vi "ReadChannelStatusFPGA.vi"(7 "IEPE settling blocks":i32=20, 8 "error in":errorcluster, 10 "Wfm Data":waveform(sgl)[](array[waveform]), 11 "Dynamic FPGA VI Reference":T1) -> (0 "error out":errorcluster, 2 "Wfm Data":waveform(sgl)[](array[waveform]), 3 "Dynamic FPGA VI Reference":T1)   [LabVIEW 2015]
doc: "This VI sets the host application's data buffer size, which is critical for maximum data throughput. This buffer is responsible for receiving data coming from the FPGA DMA FIFO. For the continuous case the buffer size should be many times larger than your read size. In the finite case, the timing VIs automatically call this VI and set the buffer size equal to the number of samples in the acquisition."
uses:
  <vilib>/addons/InsightCM/Devices/Shared/cRIOWfmAcq/subVIs/RIO Wfm Cust Ctrls/rwfm_DynamicFPGAref2.ctl
  <vilib>/addons/InsightCM/Devices/Shared/cRIOWfmAcq/subVIs/stretchState.ctl
  <vilib>/rvi/interface/nirviReadWriteControl/nirviReadWriteControl.xnode
  <vilib>/addons/InsightCM/Devices/Shared/cRIOWfmAcq/cRIOWfmLib.lvlib
  NiFpgaLv.dll
  <vilib>/Utility/error.llb/Error Cluster From Error Code.vi
  <vilib>/rvi/interface/Simulation/niFpgaSimulationCallBeginRW.vi
  <vilib>/rvi/errors/niLvFpgaAdjustHostInterfaceError.vi
  <vilib>/addons/InsightCM/Utilities/ChannelStatus/ChannelStatus.lvlib
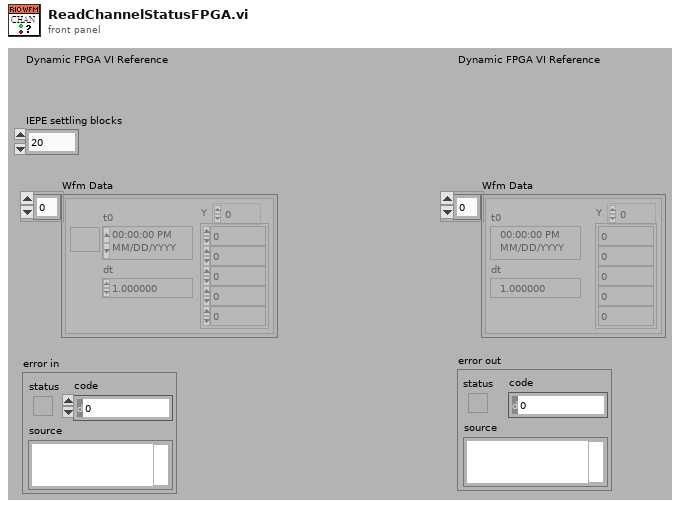
[diagram p1: front panel]
types:
  T1 = typedef "cRIOWfmLib.lvlib/rwfm_DynamicFPGAref2.ctl" = refnum<k20>
  T2 = typedef "cRIOWfmLib.lvlib/stretchState.ctl" = cluster{"input":bool, "output":bool, "pulse count":i32}
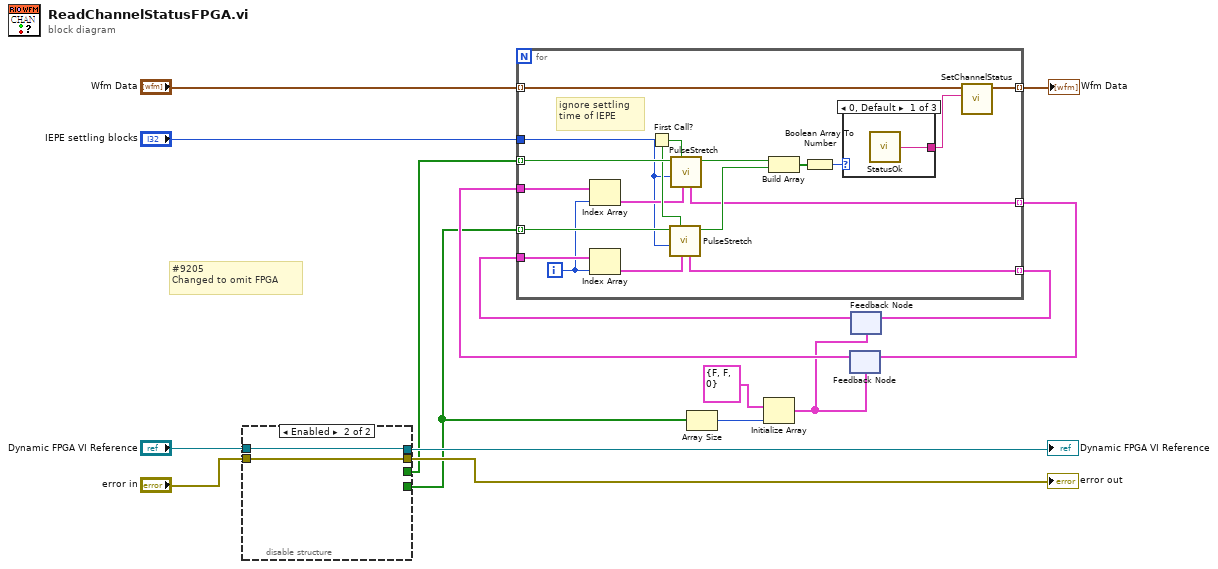
[diagram p0: block diagram]
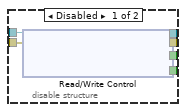
[diagram p2: hidden frame]
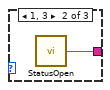
[diagram p3: hidden frame]
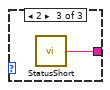
[diagram p4: hidden frame]
diagram:
  # "#9205\nChanged to omit FPGA"
  n1 = disable-structure shown="Enabled" {
    disable-tunnel: "Dynamic FPGA VI Reference" -> [w22 w24]
    disable-tunnel: "error in" -> [w21 w23]
    disable-tunnel: [w20 w24] -> w14
    disable-tunnel: [w19 w23] -> w13
    disable-tunnel: [w18 _] -> w11
    disable-tunnel: [w17 _] -> w5
    frame Disabled {
      n2 = xnode "Read/Write Control"("FPGA VI Reference In"=w22, "error in"=w21) -> ("FPGA VI Reference Out"=w20:T1, "error out"=w19:errorcluster, "Open Loop Chan Array"=w18:bool[], "Short Circuit Chan Array"=w17:bool[])
    }
    frame Enabled {
    }
  }
  "error out" <- w13
  "Dynamic FPGA VI Reference" <- w14
  n3 = Array Size(array=w5) -> (size(s)=w4:i32)
  n4 = Initialize Array(T2 {"input"=FALSE, "output"=FALSE, "pulse count"=0} ("element"), w4) -> (w2:T2[])
  n5 = feedback #1(w2) -> (w6:T2[])
  n6 = feedback #2(w2) -> (w8:T2[])
  n7 = for {
    tunnel: "Wfm Data" -> [w26] mode=indexing
    tunnel: w11 -> [w42] mode=indexing
    tunnel: w5 -> [w40] mode=indexing
    tunnel: [w25] -> w10 mode=indexing
    tunnel: [w37] -> w9 mode=indexing
    tunnel: [w36] -> w7 mode=indexing
    tunnel: w8 -> [w35]
    tunnel: w6 -> [w33]
    tunnel: "IEPE settling blocks" -> [w30]
    i -> [w31]
    # "ignore settling \ntime of IEPE"
    n8 = Index Array(array=w33, index=w31) -> (element=w32:T2)
    n9 = Index Array(array=w35, index=w31) -> (element=w34:T2)
    n10 = First Call?() -> (First Call?: T/F=w38:bool)
    n11 = call <vilib>:"PulseStretch.vi"("state in"=w34, "Reset"=w38, "Pulse Width"=w30, "Input"=w40) -> ("Output"=w39:bool, "state out"=w37:T2)  [unwired: 6 in]
    n12 = call <vilib>:"PulseStretch.vi"("state in"=w32, "Reset"=w38, "Pulse Width"=w30, "Input"=w42) -> ("Output"=w41:bool, "state out"=w36:T2)  [unwired: 6 in]
    n13 = Build Array(w41, w39) -> (w29:bool[])
    n14 = Boolean Array To Number(Boolean array=w29) -> (number=w28:u32)
    n15 = case shown="0, Default" w28 {
      tunnel: [w43 w44 w45] -> w27
      frame 0, Default {
        n16 = call <vilib>:"StatusOk.vi"() -> ("status"=w43:string)  [unwired: 5 in]
      }
      frame 1, 3 {
        n17 = call <vilib>:"StatusOpen.vi"() -> ("status"=w44:string)  [unwired: 5 in]
      }
      frame 2 {
        n18 = call <vilib>:"StatusShort.vi"() -> ("status"=w45:string)  [unwired: 5 in]
      }
    }
    n19 = call <vilib>:"SetChannelStatus.vi"("Channel Status"=w27, "Waveform in"=w26) -> ("Waveform out"=w25:waveform(sgl))  [unwired: 8 in, 1 out]
  }
  "Wfm Data" <- w10
  n20 = feedback-in #1(w7) -> ()
  n21 = feedback-in #2(w9) -> ()
